vi "AM.vi"() -> ()   [LabVIEW 2014]
panel:
  out "carrier":dynamicdata(graph)
  out "message":dynamicdata(graph)
  in  "stop":bool
  out "Waveform Graph":dynamicdata(graph)
  in  "Amplitude":dbl=1.0
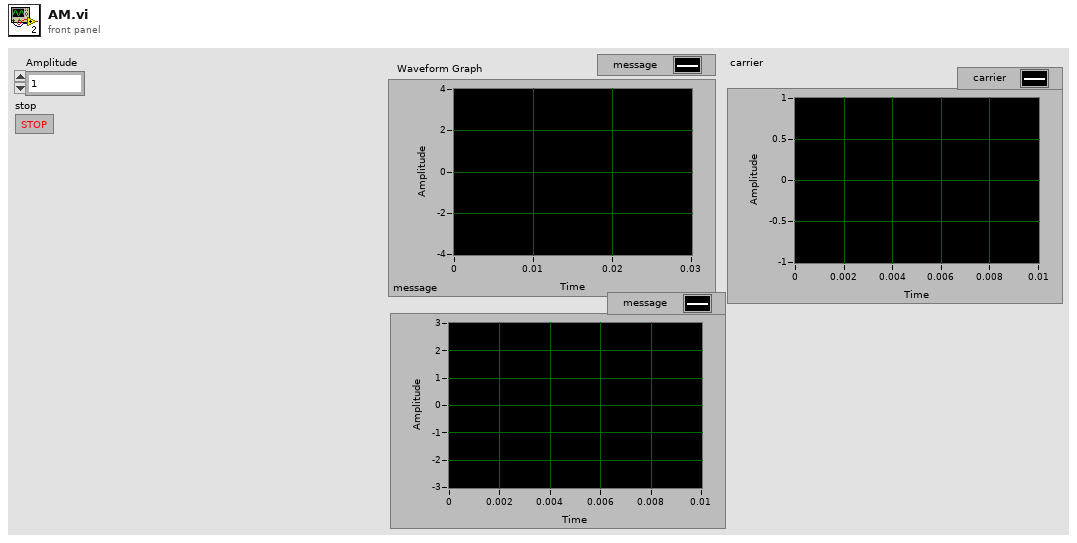
[diagram p1: front panel]
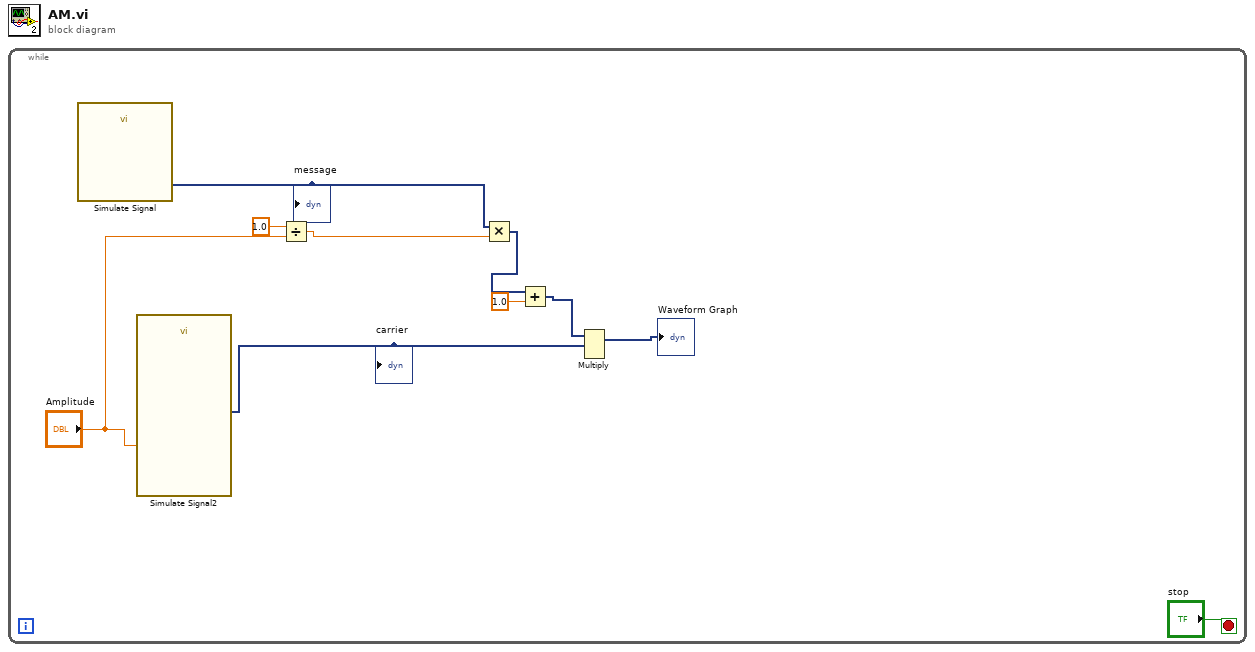
[diagram p0: block diagram]
diagram:
  n1 = while {
    stop <- "stop" stop-if-true
    n2 = call "Simulate Signal"() -> ("message"=w7:dynamicdata)  [unwired: 14 in, 1 out]
    "message" <- w7
    n3 = call "Simulate Signal2"("Amplitude"="Amplitude") -> ("carrier"=w2:dynamicdata)  [unwired: 13 in, 1 out]
    "carrier" <- w2
    n4 = Divide(x=1.0, y="Amplitude") -> (x/y=w8:dbl)
    n5 = Multiply(x=w7, y=w8) -> (x*y=w6:dynamicdata)
    n6 = Add(x=w6, y=1.0) -> (x+y=w3:dynamicdata)
    n7 = Multiply(1:w2, 2:w3) -> (0:→"Waveform Graph":dynamicdata)  [unwired: 1 in, 1 out]
  }
